vi "Align Error Message.vi"(11 "message in":string) -> (3 "message out":string)   [LabVIEW 2021, in "Game of Life.lvlib"]
doc: "This VI replaces all the 'End of Line' and 'Line Feed' constants in the given error message with the 'Space' constant."
uses:
  Game of Life.lvlib
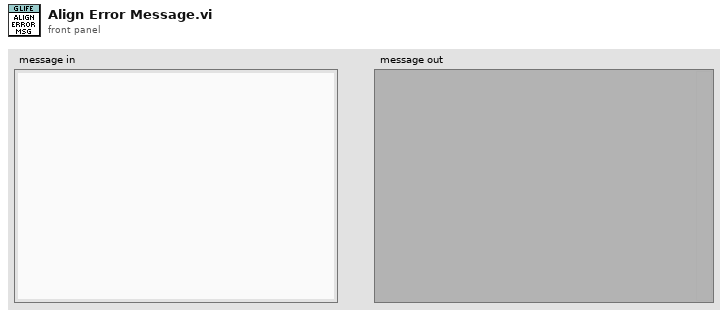
[diagram p1: front panel]
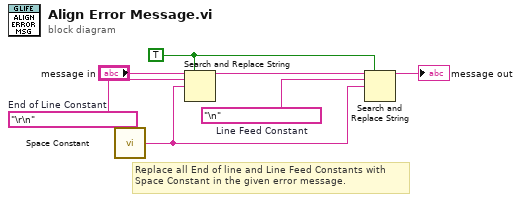
[diagram p0: block diagram]
diagram:
  w6 = "\r\n"  # End of Line Constant
  w5 = "\n"  # Line Feed Constant
  w3 = TRUE ("replace all? (F)")
  # "Replace all End of line and Line Feed Constants with\nSpace Constant in the given error message."
  n1 = call <vilib>:"Space Constant.vi"() -> ("String"=w1:string)
  n2 = Search and Replace String(replace all?=w3, input string="message in", search string=w6, replace string=w1) -> (result string=w7:string)  [unwired: 4 in, 3 out]
  n3 = Search and Replace String(replace all?=w3, input string=w7, search string=w5, replace string=w1) -> (result string=→"message out":string)  [unwired: 4 in, 3 out]
